vi "Get JS Variables For Picture Ring.vi"(8 "error in (no error)":errorcluster, 10 "Ring Images In":variant, 11 "Ring in":refnum<vi>) -> (0 "error out":errorcluster, 2 "Ring Images Out":variant, 3 "Ring Image Variable Name":string)   [LabVIEW 2017, in "Front Panel Publisher.lvlib" / "Select.lvclass"]
uses:
  Select.lvclass
  <vilib>/wsapi/NI_WebServices.lvlib
  Front Panel Publisher.lvlib
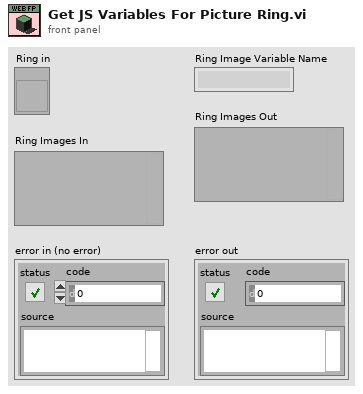
[diagram p1: front panel]
types:
  T1 = enum32{"Text Ring", "Pict Ring", "Text and Pict Ring"}
  T2 = typedef "LVRectTypeDef.ctl" = cluster{"Left":i16, "Top":i16, "Right":i16, "Bottom":i16}
  T3 = cluster{"NumItems":u32, "Size Out":cluster{"Width":u32, "Height":u32}}
  T4 = typedef "imagedata.ctl" = cluster{"image type":i32, "image depth":i32, "image":u8[], "mask":u8[], "colors":u32[], "Rectangle":cluster{"left":i16, "top":i16, "right":i16, "bottom":i16}}
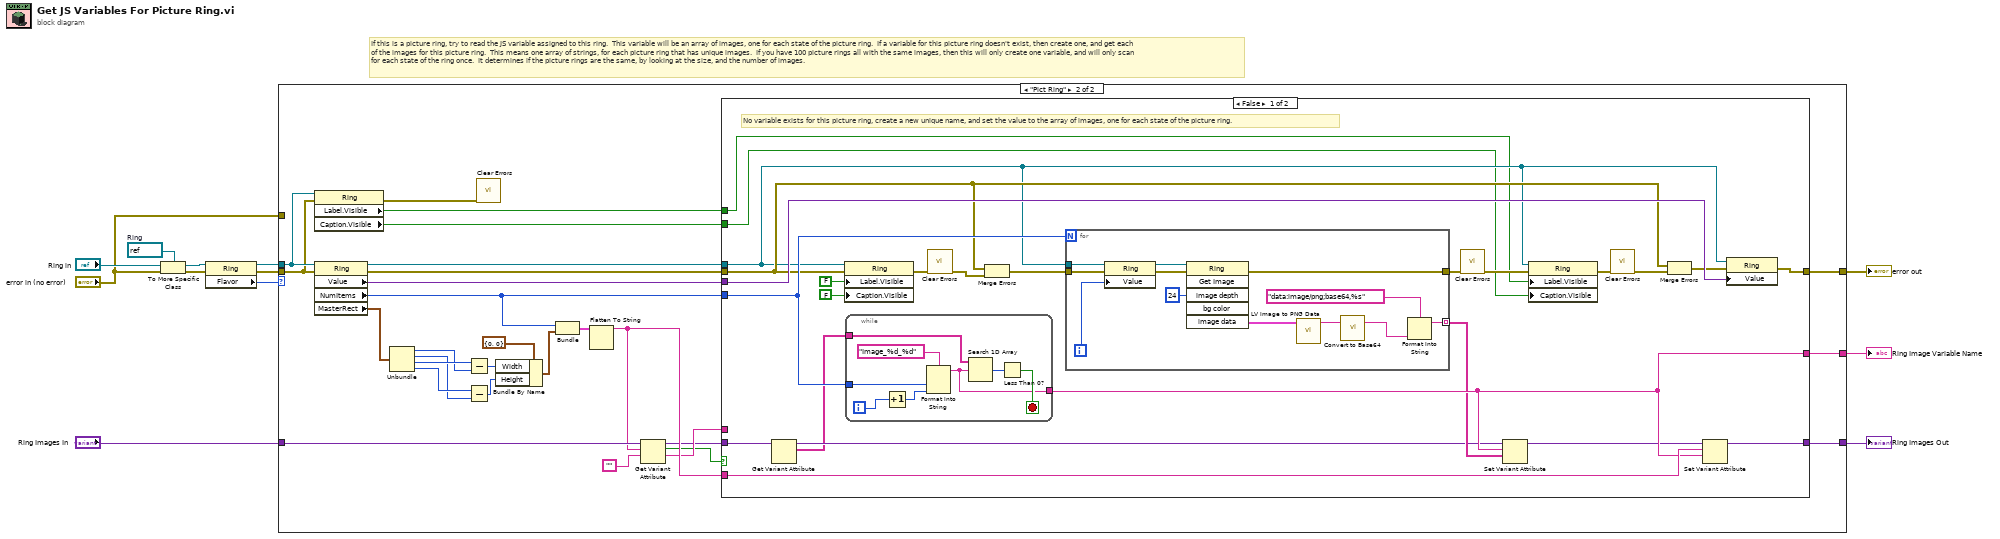
[diagram p0: block diagram]
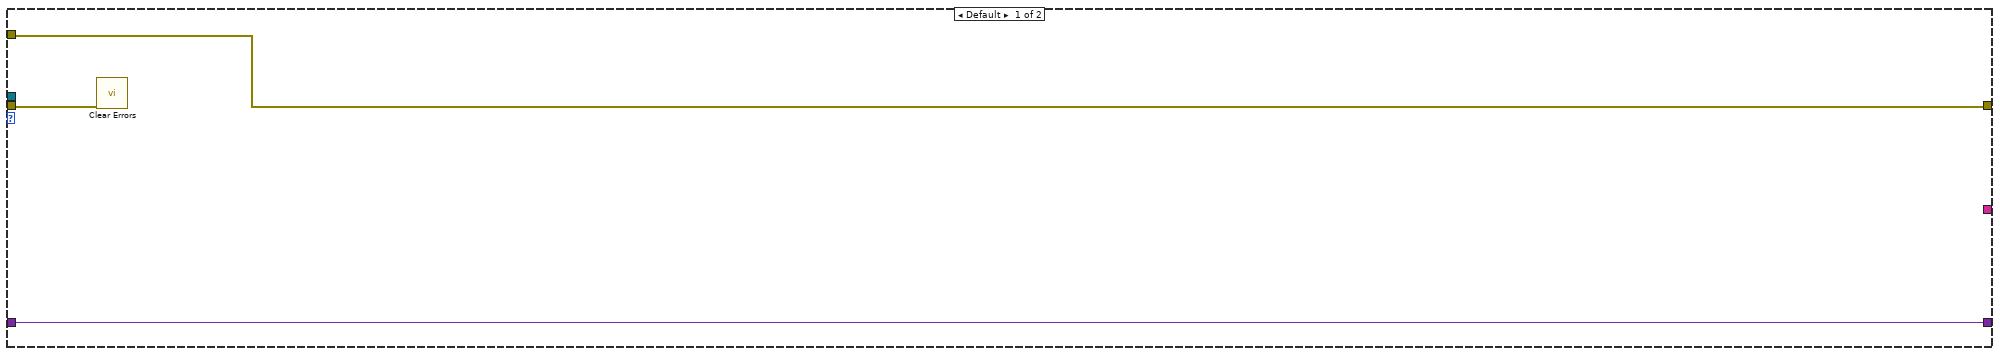
[diagram p2: hidden frame]
diagram:
  w5 = refnum<vi> refnum  # Ring
  # "If this is a picture ring, try to read the JS variable assigned to this ring.  This variable will be an array of images, one for each state of the picture ring.  If a variable for this picture ring doesn't exist, then create one, and get each of the images for this picture ring.  This means one array of strings, for each picture ring that has unique images.  If you have 100 picture rings all with the same images, then this will only create one variable, and will only scan for each state of the ring once.  It determines if the picture rings are the same, by looking at the size, and the number of images."
  n1 = To More Specific Class(target class=w5, reference="Ring in", error in="error in (no error)") -> (specific class reference=w1:refnum<vi>, error out=w2:errorcluster)
  n2 = property on="Property Node" class="Ring"(reference=w1, error in=w2) -> (reference out=w11:refnum<vi>, error out=w10:errorcluster, "Flavor"=w12:T1)
  n3 = case shown="\"Pict Ring\"" w12 {
    tunnel: w11 -> [_ w35]
    tunnel: w10 -> [w13 w34]
    tunnel: [w14 w43] -> w8
    tunnel: [w15 w42] -> w7
    tunnel: "Ring Images In" -> [w15 w30]
    tunnel: [_ w36] -> w6
    tunnel: "error in (no error)" -> [w14 _]
    frame Default {
      n4 = call <vilib>:"Clear Errors.vi"("error in (no error)"=w13) -> ()  [unwired: 5 in, 2 out]
    }
    frame "Pict Ring" {
      n5 = property on="Property Node" class="Ring"(reference=w35, error in=w34) -> (error out=w31:errorcluster, "Label.Visible"=w33:bool, "Caption.Visible"=w32:bool)  [unwired: 1 out]
      n6 = property on="Property Node" class="Ring"(reference=w35, error in=w34) -> (reference out=w40:refnum<vi>, error out=w39:errorcluster, "Value"=w41:variant, "NumItems"=w37:u32, "MasterRect"=w18:T2)
      n7 = Unbundle(w18) -> ("Left"=w24:i16, "Top"=w20:i16, "Right"=w25:i16, "Bottom"=w21:i16)
      n8 = Subtract(x=w25, y=w24) -> (x-y=w22:i16)
      n9 = Subtract(x=w21, y=w20) -> (x-y=w19:i16)
      n10 = call <vilib>:"Clear Errors.vi"("error in (no error)"=w31) -> ()  [unwired: 5 in, 2 out]
      n11 = Bundle By Name(cluster=cluster{"Width":u32, "Height":u32} {"Width"=0, "Height"=0} ("Size Out"), "Width"=w22, "Height"=w19) -> (w17:cluster{"Width":u32, "Height":u32})
      n12 = Bundle("NumItems"=w37, "Size Out"=w17) -> (w38:T3)  [unwired: 1 in]
      n13 = Flatten To String(anything=w38) -> (data string=w29:string)  [unwired: 3 in, 2 out]
      n14 = Get Variant Attribute(Variant=w30, name=w29, default value (empty Variant)="") -> (duplicate Variant=w26:variant, found=w16:bool, value=w27:string)  [unwired: 1 in, 1 out]
      n15 = case shown="False" w16 {
        tunnel: w41 -> [w68 _]
        tunnel: [w65 w91] -> w43
        tunnel: w37 -> [w64 _]
        tunnel: w40 -> [w54 _]
        tunnel: w39 -> [w59 w91]
        tunnel: w29 -> [w51 _]
        tunnel: [w50 w90] -> w42
        tunnel: w26 -> [w46 w90]
        tunnel: [w49 w89] -> w36
        tunnel: w27 -> [_ w89]
        tunnel: w33 -> [w53 _]
        tunnel: w32 -> [w52 _]
        frame False {
          # "No variable exists for this picture ring, create a new unique name, and set the value to the array of images, one for each state of the picture ring."
          n16 = Get Variant Attribute(Variant=w46) -> (duplicate Variant=w45:variant, names=w44:string[])  [unwired: 3 in, 2 out]
          n17 = property on="Property Node" class="Ring"(reference=w54, error in=w59, "Label.Visible"=FALSE, "Caption.Visible"=FALSE) -> (error out=w61:errorcluster)  [unwired: 1 out]
          n18 = while {
            tunnel: w64 -> [w75]
            tunnel: w44 -> [w72]
            tunnel: [w69] -> w49
            i -> [w74]
            stop <- w70 stop-if-true
            n19 = Increment(x=w74) -> (x+1=w73:i32)
            n20 = Format Into String(format string="Image_%d_%d", w75, w73) -> (resulting string=w69:string)  [unwired: 2 in, 1 out]
            n21 = Search 1D Array(1D array=w72, element=w69) -> (index of element=w71:i32)  [unwired: 1 in]
            n22 = Less Than 0?(x=w71) -> (x < 0?=w70:bool)
          }
          n23 = call <vilib>:"Clear Errors.vi"("error in (no error)"=w61) -> ("error out"=w60:errorcluster)  [unwired: 5 in, 1 out]
          n24 = Merge Errors(w59, w60) -> (w58:errorcluster)
          n25 = for {
            N: w64 -> [_]
            tunnel: w58 -> [w88]
            tunnel: w54 -> [w85]
            tunnel: [w83] -> w66
            tunnel: [w77] -> w48 mode=indexing
            i -> [w78]
            n26 = property class="Ring"(reference=w85, error in=w88, "Value"=w78) -> (reference out=w84:refnum<vi>, error out=w86:errorcluster)
            n27 = invoke on="Invoke Node" class="Ring" method="Get Image"(reference=w84, error in=w86, "image depth"=24 ("Image Depth")) -> (error out=w83:errorcluster, "image data"=w79:T4)  [unwired: 3 in, 4 out]
            n28 = call <vilib>:"LV Image to PNG Data.vi"("image data"=w79) -> ("png data"=w80:string)  [unwired: 9 in, 1 out]
            n29 = call "Convert to Base64.vi"("String"=w80) -> ("Base64 String"=w82:string)  [unwired: 2 in]
            n30 = Format Into String(format string="data:image/png;base64,%s" ("string"), w82) -> (resulting string=w77:string)  [unwired: 2 in, 1 out]
          }
          n31 = call <vilib>:"Clear Errors.vi"("error in (no error)"=w66) -> ("error out"=w57:errorcluster)  [unwired: 5 in, 1 out]
          n32 = Set Variant Attribute(Variant=w45, name=w49, value=w48) -> (Variant out=w47:variant)  [unwired: 1 in, 2 out]
          n33 = property on="Property Node" class="Ring"(reference=w54, error in=w57, "Label.Visible"=w53, "Caption.Visible"=w52) -> (error out=w56:errorcluster)  [unwired: 1 out]
          n34 = call <vilib>:"Clear Errors.vi"("error in (no error)"=w56) -> ("error out"=w55:errorcluster)  [unwired: 5 in, 1 out]
          n35 = Merge Errors(w59, w55) -> (w67:errorcluster)
          n36 = Set Variant Attribute(Variant=w47, name=w51, value=w49) -> (Variant out=w50:variant)  [unwired: 1 in, 2 out]
          n37 = property on="Property Node" class="Ring"(reference=w54, error in=w67, "Value"=w68) -> (error out=w65:errorcluster)  [unwired: 1 out]
        }
        frame True {
          # "Variable already exists, just pass it out."
        }
      }
    }
  }
  "error out" <- w8
  "Ring Image Variable Name" <- w6
  "Ring Images Out" <- w7
